vi "input.vi"(3 "error in (no error)":errorcluster, 4 "commando":string, 5 "VISA in":refnum<visa-resource-name>) -> (0 "error out":errorcluster, 1 "DEBUG":string, 2 "VISA out":refnum<visa-resource-name>)   [LabVIEW 2022 SP3]
uses:
  <vilib>/Instr/_visa.llb/VISA Configure Serial Port (Instr).vi
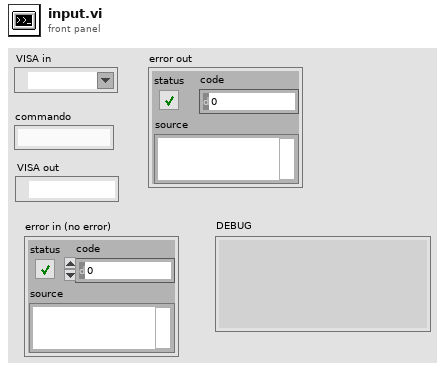
[diagram p1: front panel]
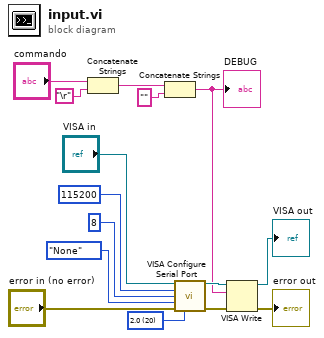
[diagram p0: block diagram]
diagram:
  w15 = u16 20 items=["Eli"=64, "1.0"=10, "1.5"=15, "2.0"=20] ("stop bits (10: 1 bit)")
  n1 = Concatenate Strings("commando", "\r") -> (w3:string)
  n2 = Concatenate Strings(w3, "" ("string")) -> (w1:string)
  "DEBUG" <- w1
  n3 = call-poly "VISA Configure Serial Port"("VISA resource name"="VISA in", "baud rate (9600)"=u32 115200, "data bits (8)"=u16 8, "parity (0:none)"=enum16{"None", "Odd", "Even", "Mark", "Space"}."None", "error in (no error)"="error in (no error)", "stop bits (10: 1 bit)"=w15) -> ("VISA resource name out"=w9:refnum<visa-resource-name>, "error out"=w10:errorcluster)  [unwired: 8 in]
  n4 = VISA Write(VISA resource name=w9, write buffer=w1, error in (no error)=w10) -> (VISA resource name out=→"VISA out":refnum<visa-resource-name>, error out=→"error out":errorcluster)  [unwired: 1 out]
